vi "AC Bitfile pointer.vi"(11 "Target":T2) -> (0 "error out":errorcluster, 3 "FGPA Ref":T1)   [LabVIEW 2013]
uses:
  <vilib>/userdefined/High Color/nirio_resource_hc.ctl
  FPGA Refs/FPGA Ref.ctl
  <vilib>/FPGAPlugInAG/PXIe-7966R/niLvFpga_Open_PXIe-7966R.vi
  <vilib>/rvi/interface/common/dynamic/niFpgaDynamicAddResources.vi
  <vilib>/rvi/interface/nirviOpenFPGA/nirviOpenFPGA.xnode
  FPGA DAQ-AC.lvbitx
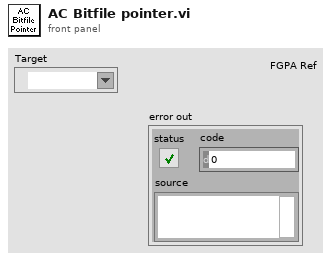
[diagram p1: front panel]
types:
  T1 = typedef "FPGA Ref.ctl" = refnum<k20>
  T2 = typedef "nirio_resource_hc.ctl" = tag
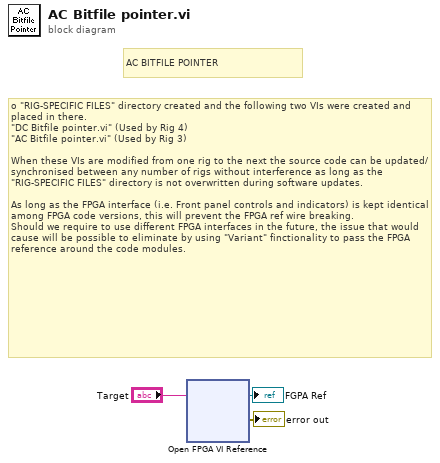
[diagram p0: block diagram]
diagram:
  # "AC BITFILE POINTER"
  # "o\t\"RIG-SPECIFIC FILES\" directory created and the following two VIs were created and placed in there. \n\"DC Bitfile pointer.vi\" (Used by Rig 4)\n\"AC Bitfile pointer.vi\" (Used by Rig 3)\n\nWhen these VIs are modified from one rig to the next the source code can be updated/synchronised between any number of rigs without interference as long as the \"RIG-SPECIFIC FILES\" directory is not overwritten during software updates.\n\nAs long as the FPGA interface (i.e. Front panel controls and indicators) is kept identical among FPGA code versions, this will prevent the FPGA ref wire breaking.\nShould we require to use different FPGA interfaces in the future, the issue that would cause will be possible to eliminate by using \"Variant\" finctionality to pass the FPGA reference around the code modules."
  n1 = xnode ("Open FPGA VI Reference")("resource name"="Target") -> ("FPGA VI Reference Out"=→"FGPA Ref":refnum<k20>, "error out"=→"error out":errorcluster)  [unwired: 1 in]
